vi "event.create_programmatic.path.vi"() -> (3 "path":string)   [LabVIEW 2020, in "Nominal Client.lvclass"]
uses:
  Nominal Client.lvclass
  Nominal Client.lvclass/Nominal Client.ctl
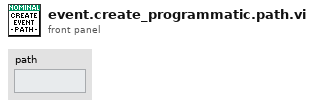
[diagram p1: front panel]
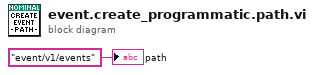
[diagram p0: block diagram]
diagram:
  "path" <- "event/v1/events" ("path")
